vi "SetRecordLength.vi"(8 "error in (no error)":errorcluster, 10 "Samples per 5782 record":i32, 11 "ScopeBase In":refnum<class "ScopeBase.lvclass">) -> (0 "error out":errorcluster, 3 "ScopeBase Out":refnum<class "ScopeBase.lvclass">)   [LabVIEW 2018, in "ScopeBase.lvclass"]
uses:
  ScopeBase.lvclass
  ScopeBase.lvclass/ScopeBase.ctl
  <vilib>/Utility/error.llb/Error Cluster From Error Code.vi
  <vilib>/rvi/errors/niLvFpgaAdjustHostInterfaceError.vi
  <vilib>/rvi/interface/nirviReadWriteControl/nirviReadWriteControl.xnode
  FpgaRef/FpgaRefBase/Common FPGA ref.ctl
  FpgaRef/FpgaRefBase/FpgaRefBase.lvclass
  NiFpgaLv.dll
  <vilib>/rvi/interface/Simulation/niFpgaSimulationCallBeginRW.vi
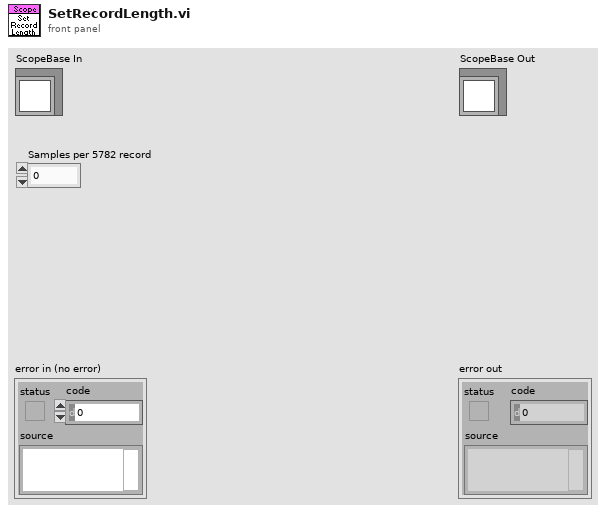
[diagram p1: front panel]
types:
  T1 = typedef "Common FPGA ref.ctl" = refnum<k20>
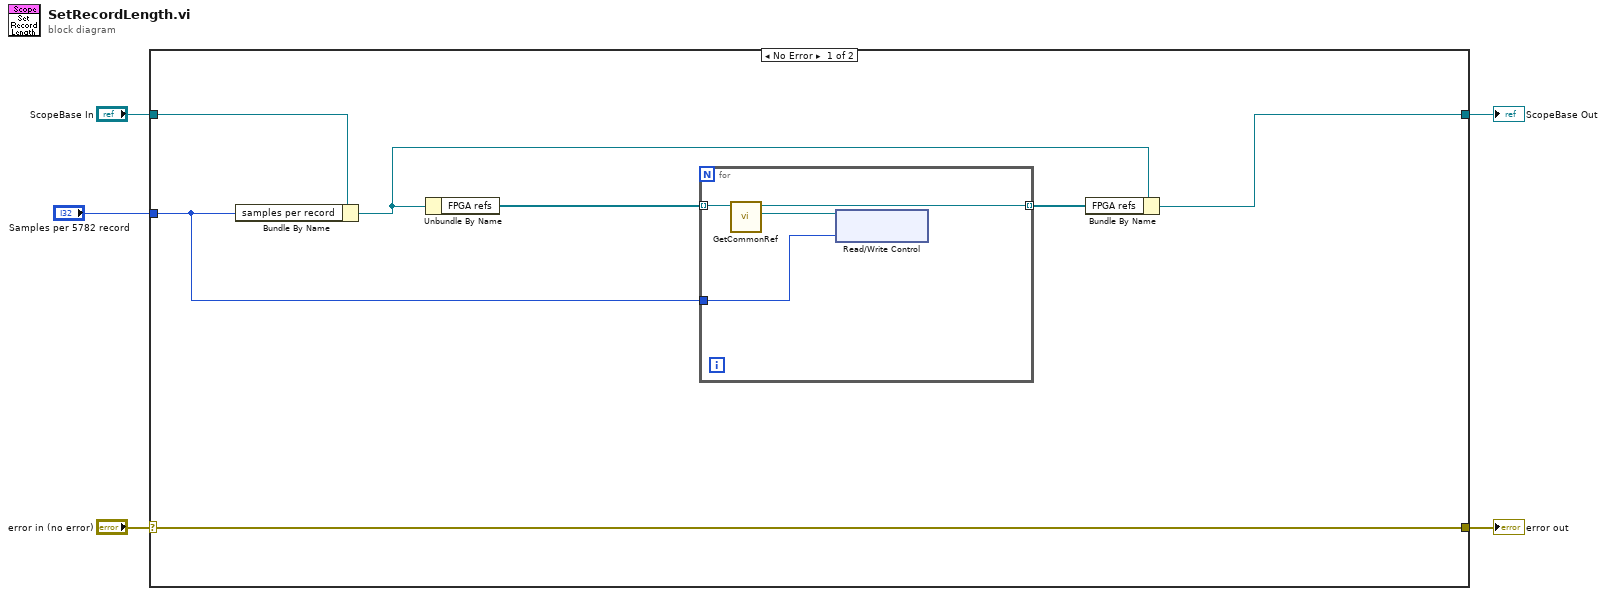
[diagram p0: block diagram]
diagram:
  n1 = case shown="No Error" "error in (no error)" {
    selector: "error in (no error)" -> [w12 w18]
    tunnel: [w12 w18] -> w3
    tunnel: [w6 w17] -> w4
    tunnel: "ScopeBase In" -> [w11 w17]
    tunnel: "Samples per 5782 record" -> [w7 _]
    frame No Error {
      n2 = Bundle By Name(cluster=w11, "samples per record"=w7) -> (w8:refnum<class "ScopeBase.lvclass">)
      n3 = Unbundle By Name(w8) -> ("FPGA refs"=w10:refnum<class "FpgaRefBase.lvclass">[])
      n4 = for {
        tunnel: w7 -> [w16]
        tunnel: w10 -> [w15] mode=indexing
        tunnel: [w13] -> w9 mode=indexing
        n5 = call-dynamic "GetCommonRef.vi"("FpgaRefBase in"=w15) -> ("Common ref"=w14:T1, "FpgaRefBase out"=w13:refnum<class "FpgaRefBase.lvclass">)  [unwired: 8 in, 1 out]
        n6 = xnode "Read/Write Control"("FPGA VI Reference In"=w14, "Record length"=w16) -> ()  [unwired: 1 in, 2 out]
      }
      n7 = Bundle By Name(cluster=w8, "FPGA refs"=w9) -> (w6:refnum<class "ScopeBase.lvclass">)
    }
    frame Error {
    }
  }
  "error out" <- w3
  "ScopeBase Out" <- w4
